vi "Dispense.vi"(8 "Error In":errorcluster, 10 "Selection":bool[](array[boolean]), 11 "Money":i32) -> (0 "Error Out":errorcluster)   [LabVIEW 2020]
doc: "This VI is dialog program which simulate process of dispensing products and change by vending machine. Needs inserted money value and \"choice array\". Comments in Polish."
panel:
  in  "Stop":bool
  out "Info":string
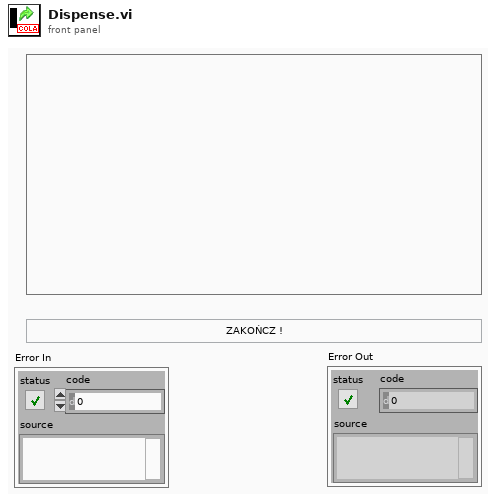
[diagram p1: front panel]
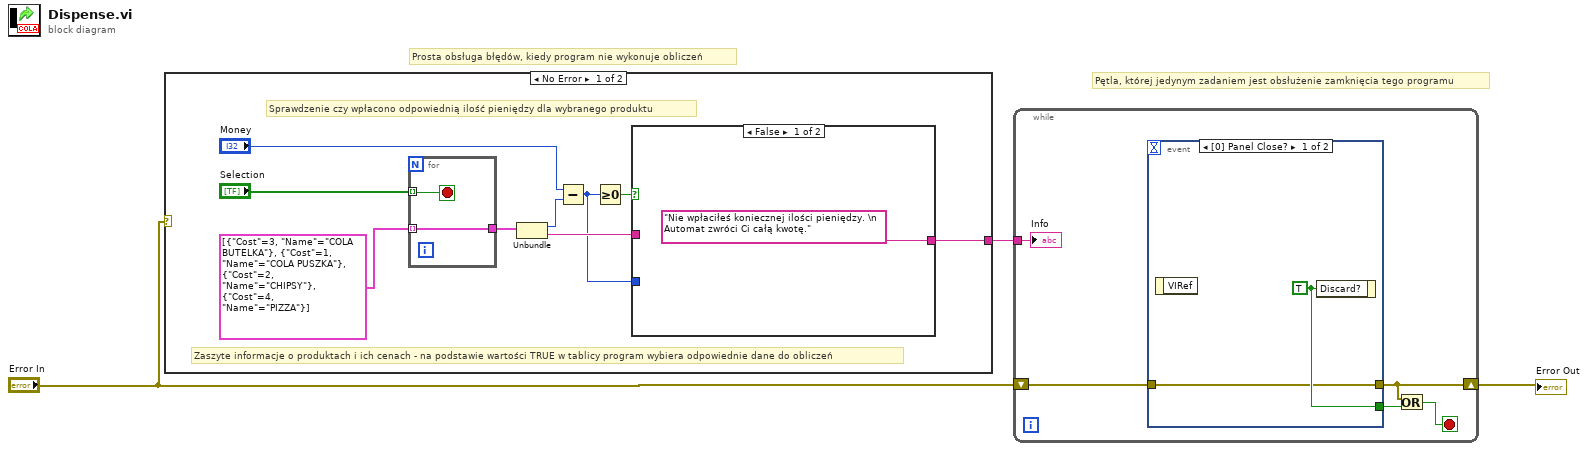
[diagram p0: block diagram]
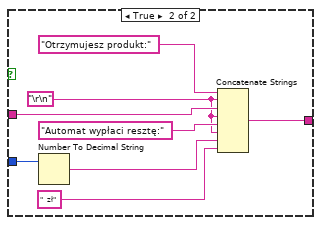
[diagram p2: hidden frame]
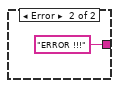
[diagram p3: hidden frame]
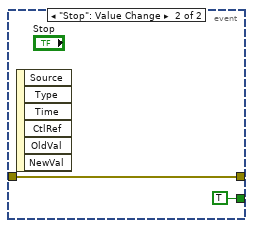
[diagram p4: hidden frame]
diagram:
  # "Pętla, której jedynym zadaniem jest obsłużenie zamknięcia tego programu"
  # "Prosta obsługa błędów, kiedy program nie wykonuje obliczeń"
  n1 = case shown="No Error" "Error In" {
    tunnel: [w4 "ERROR !!!"] -> w2
    frame No Error {
      # "Sprawdzenie czy wpłacono odpowiednią ilość pieniędzy dla wybranego produktu"
      # "Zaszyte informacje o produktach i ich cenach - na podstawie wartości TRUE w tablicy program wybiera odpowiednie dane do obliczeń"
      n2 = for {
        tunnel: "Selection" -> [w23] mode=indexing
        tunnel: cluster{"Cost":i32, "Name":string}[] [{"Cost"=3, "Name"="COLA BUTELKA"}, {"Cost"=1, "Name"="COLA PUSZKA"}, {"Cost"=2, "Name"="CHIPSY"}, {"Cost"=4, "Name"="PIZZA"}] -> [w22] mode=indexing
        tunnel: [w22] -> w10
        stop <- w23 stop-if-true
      }
      n3 = Unbundle(w10) -> ("Cost"=w9:i32, "Name"=w6:string)
      n4 = Subtract(x="Money", y=w9) -> (x-y=w5:i32)
      n5 = Greater Or Equal To 0?(x=w5) -> (x >= 0?=w7:bool)
      n6 = case shown="False" w7 {
        tunnel: w6 -> [_ w19]
        tunnel: ["Nie wpłaciłeś koniecznej ilości pieniędzy. \n Automat zwróci Ci całą kwotę." w14] -> w4
        tunnel: w5 -> [_ w17]
        frame False {
        }
        frame True {
          w18 = "\r\n"
          n7 = Number To Decimal String(number=w17) -> (decimal integer string=w16:string)  [unwired: 1 in]
          n8 = Concatenate Strings("Otrzymujesz produkt:", w18, w19, w18, "Automat wypłaci resztę:", w18, w16, "  zł" ("string")) -> (w14:string)
        }
      }
    }
    frame Error {
    }
  }
  n9 = while {
    tunnel: w2 -> [w26]
    shift-right: [w28] -> w1
    shift-left: "Error In" -> [w29]
    stop <- w27 stop-if-true
    n10 = event shown="[0] Panel Close?" {
      selector: _ -> [_ _]
      dyn-events: _ -> [_ _]
      timeout: _ -> [_ _]
      tunnel: w29 -> [w30 w33]
      tunnel: [w30 w33] -> w28
      tunnel: [w31 TRUE ("Discard?")] -> w25
      event Panel Close? {
        w31 = TRUE ("Discard?")
        n11 = event-data() -> ()  [unwired: 1 in, 1 out]
        n12 = event-data("Discard?"=w31) -> ()  [unwired: 1 in, 1 out]
      }
      event "Stop": Value Change {
        n13 = event-data() -> ()  [unwired: 1 in, 6 out]
      }
    }
    n14 = Or(x=w28, y=w25) -> (x .or. y?=w27:bool)
    "Info" <- w26
  }
  "Error Out" <- w1
